vi "Load New Launcher.vi"(7 "Plugin Loader Path Override":path, 8 "error in (no error)":errorcluster, 9 "Loader Name Override":string, 10 "Loader Load Info":T1, 11 "CIFPluginManager in":refnum<class "CIFPluginManager.lvclass">) -> (0 "error out":errorcluster)   [LabVIEW 2021, in "CIFPluginManager.lvclass"]
uses:
  CIFPluginManager.lvclass
  typedef/Loader Load Command.ctl
  typedef/Loader Type.ctl
  CIFPluginManager.lvclass/CIFPluginManager.ctl
  <vilib>/CIF Foundation/CIF Core/CIFUtilities/CIFConfigurationFile/typedef/Location Type.ctl
  <vilib>/CIF Foundation/CIF Core/CIFCore/Common/Typedef/Errors.ctl
  <vilib>/CIF Foundation/CIF Core/CIFUtilities/CIFConfigurationFile/CIF Configuration File Location.vi
  <vilib>/CIF Foundation/CIF Utilities/Errors/Append Error Location.vi
  <vilib>/CIF Foundation/CIF Utilities/Time/System Time/LabVIEW Time to TAI Time.vi
  Engine Launch/CIF Engine Launch.lvlib
  <vilib>/CIF Foundation/CIF Utilities/Time/Time_CIF_U.lvlib
  <vilib>/CIF Foundation/CIF Core/CIFUtilities/CIFConfigurationFile/CIF Configuration File.lvlib
  <vilib>/CIF Foundation/CIF Core/CIFCore/Common/CIFCoreCommon.lvlib
  <vilib>/CIF Foundation/CIF Core/CIFUtilities/CIFLogs/CIFLogs.lvlib
  <vilib>/CIF Foundation/CIF Core/CIFUtilities/CIFLogs/Typedef/Message Type.ctl
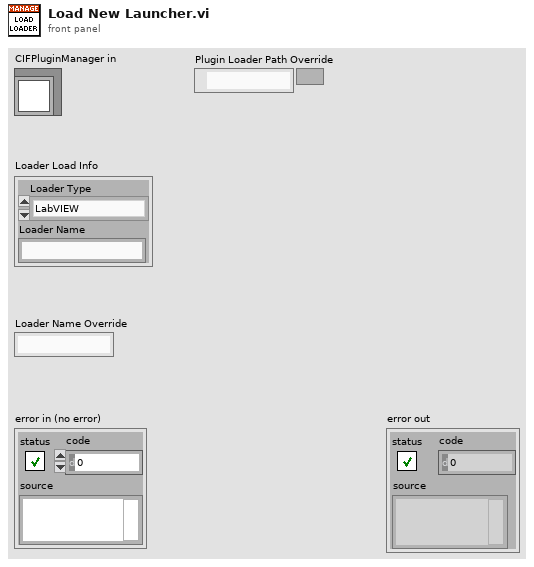
[diagram p1: front panel]
types:
  T1 = typedef "CIFPluginManager.lvclass/Loader Load Command.ctl" = cluster{"Loader Type":T2, "Loader Name":string}
  T2 = typedef "CIFPluginManager.lvclass/Loader Type.ctl" = enum16{"LabVIEW"}
  T3 = typedef "CIFPluginManager.lvclass/Loader Map.ctl" = map{string, T4}
  T4 = typedef "CIFPluginManager.lvclass/Loaders.ctl" = cluster{"Loader Type":T2, "grpc_port":i32, "pid":u32, "gRPC ID":T5, "Load Timestamp":i64, "Unloading":bool, "Ready for removal":bool, "Unload Timestamp":i64}
  T5 = typedef "grpc-lvsupport-release.lvlib/grpcId.ctl" = u64
  T6 = typedef "CIFCoreCommon.lvlib/Errors.ctl" = enum16{"Invalid Clock ID", "Long Sleep", "gRPC Server Not Found", "Config Parse", "Timestamp Wrap", "Delayed Execution", "Duplicate Channel", "Missing Channel", "Incorrect Type", "Flatten Error", "Unflatten Data", "Unique Name", "Plugin Not Found", "Plugin Type Not Found", "Plugin Version Not Found", "Manager Not Found", "Numerical Issue", "Time Jump", "Clock ID Match", "Channel Length", "Plugin Connection", "gRPC Server Connection", "PPL Name Match", "Build", "Config Log Parse", "Plugin Load", "UI Subpanel Load", "Python Name", "Invalid Name", "Unable to Change Ch Buffer", "Failed Kill", "Failed SysExec", "Function Not Implemented", "Load Timeout", "Invalid FTE", "Manager Crash"}
  T7 = typedef "CIF Configuration File.lvlib/Location Type.ctl" = enum16{"Config File", "Manager", "Protos", "Plugins", "UI Plugins", "Logs", "Orchestrations", "Loaders"}
  T8 = typedef "CIFLogs.lvlib/Message Type.ctl" = enum16{"Error", "Information", "Print Terminal", "Configuration"}
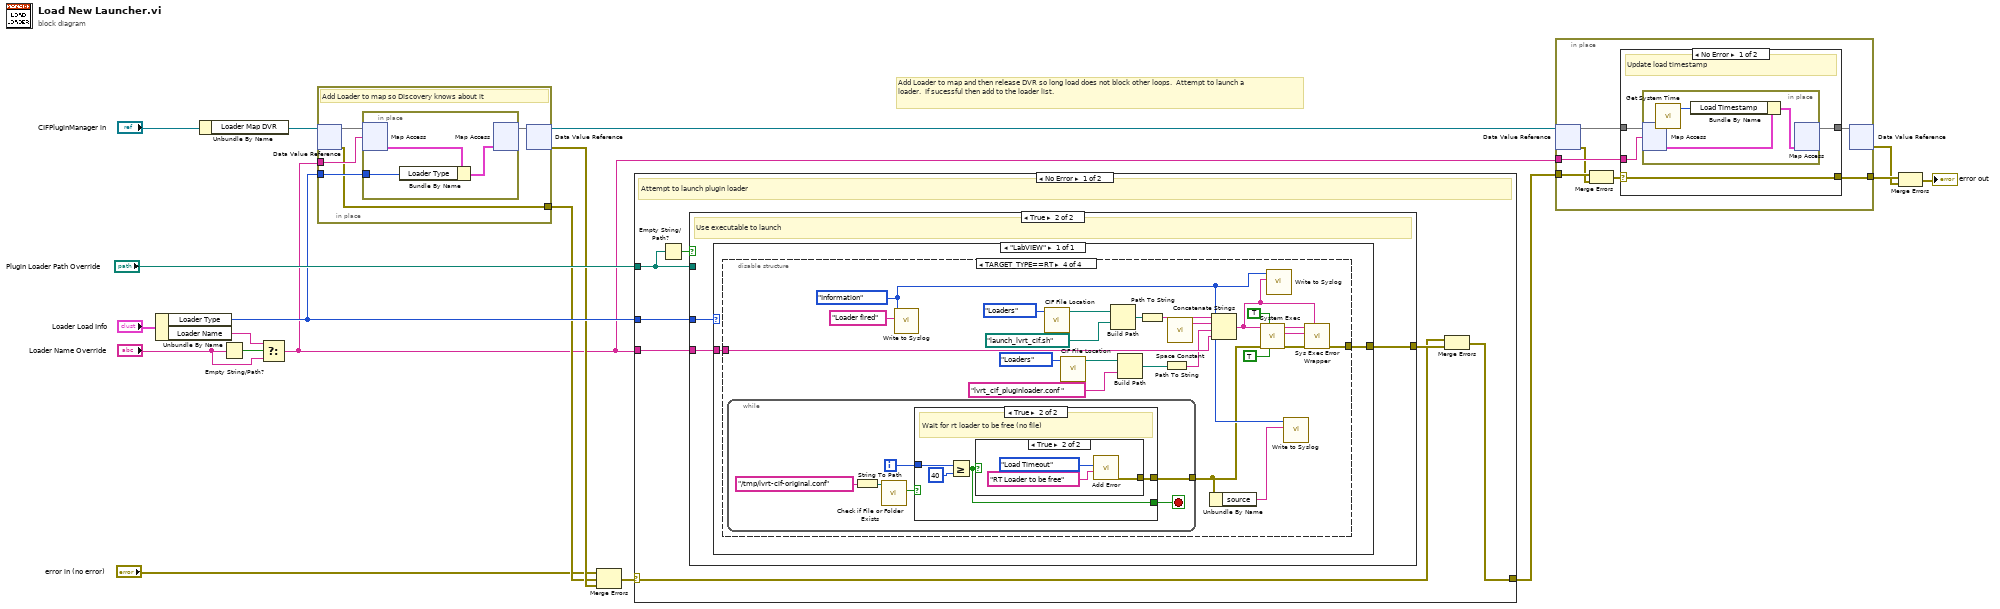
[diagram p0: block diagram]
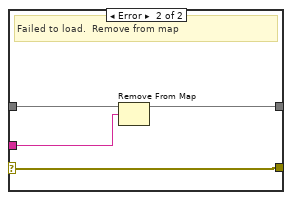
[diagram p2: hidden frame]
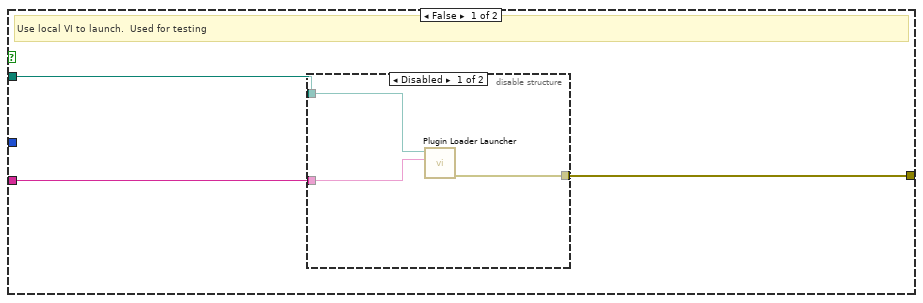
[diagram p3: hidden frame]
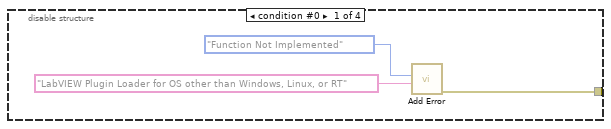
[diagram p5: hidden frame]
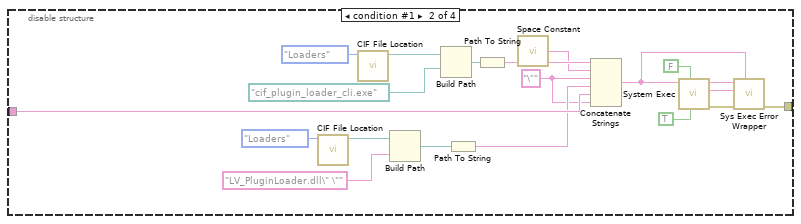
[diagram p6: hidden frame]
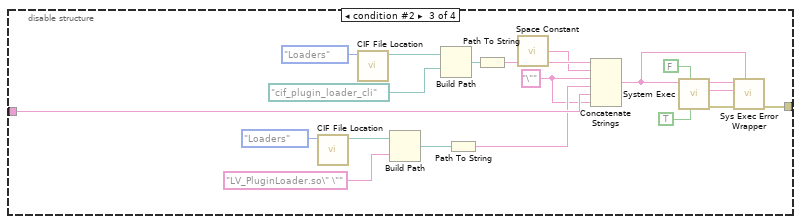
[diagram p7: hidden frame]
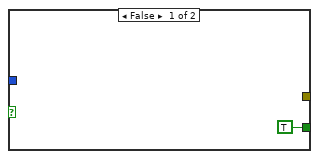
[diagram p8: hidden frame]
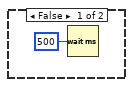
[diagram p9: hidden frame]
diagram:
  # "Add Loader to map and then release DVR so long load does not block other loops.  Attempt to launch a loader.  If sucessful then add to the loader list."
  n1 = Unbundle By Name("Loader Load Info") -> ("Loader Type"=w11:T2, "Loader Name"=w14:string)
  n2 = Unbundle By Name("CIFPluginManager in") -> ("Loader Map DVR"=w12:refnum<data-value>)
  n3 = Empty String/Path?(string/path="Loader Name Override") -> (empty?=w16:bool)
  n4 = Select(t=w14, s=w16, f="Loader Name Override") -> (s? t:f=w3:string)
  n5 = in-place {
    in-place-border: w3 -> [w22]
    in-place-border: w11 -> [w21]
    in-place-border: [w19] -> w9
    # "Add Loader to map so Discovery knows about it"
    n6 = in-place-dvr #1(w12) -> (w23:T3, w19:errorcluster)
    n7 = in-place {
      in-place-border: w21 -> [w25]
      n8 = in-place-map #2(w23, w22) -> (w26:T4)  [unwired: 1 in, 1 out]
      n9 = Bundle By Name(cluster=w26, "Loader Type"=w25) -> (w24:T4)
      n10 = in-place-map #2(w24) -> (w20:T3)  [unwired: 1 in, 2 out]
    }
    n11 = in-place-dvr #1(w20) -> (w8:refnum<data-value>, w10:errorcluster)
  }
  n12 = Merge Errors("error in (no error)", w9, w10) -> (w1:errorcluster)
  n13 = case shown="No Error" w1 {
    selector: w1 -> [w31 w126]
    tunnel: [w27 w126] -> w7
    tunnel: "Plugin Loader Path Override" -> [w30 _]
    tunnel: w3 -> [w28 _]
    tunnel: w11 -> [w33 _]
    frame No Error {
      # "Attempt to launch plugin loader"
      n14 = Empty String/Path?(string/path=w30) -> (empty?=w29:bool)
      n15 = case shown="True" w29 {
        tunnel: w30 -> [w36 _]
        tunnel: [w35 w41] -> w32
        tunnel: w28 -> [w34 w42]
        tunnel: w33 -> [_ w40]
        frame False {
          # "Use local VI to launch.  Used for testing"
          n16 = disable-structure shown="Disabled" {
            disable-tunnel: w36 -> [w39 _]
            disable-tunnel: [w38 _] -> w35
            disable-tunnel: w34 -> [w37 _]
            frame Disabled {
              n17 = call "Plugin Loader Launcher.vi"("Loader Name Override"=w37, "Plugin Loader Path Override"=w39) -> ("error out"=w38:errorcluster)  [unwired: 9 in]
            }
            frame Enabled {
            }
          }
        }
        frame True {
          # "Use executable to launch"
          n18 = case shown="\"LabVIEW\"" w40 {
            tunnel: w42 -> [w44]
            tunnel: [w43] -> w41
            frame "LabVIEW" {
              n19 = disable-structure shown="TARGET_TYPE==RT" {
                disable-tunnel: w44 -> [_ w57 w77 w100]
                disable-tunnel: [w47 w51 w71 w95] -> w43
                frame condition #0 {
                  n20 = call <vilib>:"Add Error.vi"("String to Append"="LabVIEW Plugin Loader for OS other than Windows, Linux, or RT", "Error"=Errors."Function Not Implemented") -> ("error out"=w47:errorcluster)  [unwired: 9 in]
                }
                frame condition #1 {
                  w53 = "\"" ("Loader Name Override")
                  n21 = call <vilib>:"CIF File Location.vi"("LocationType"=Location_Type."Loaders") -> ("Location"=w59:path)  [unwired: 10 in]
                  n22 = call <vilib>:"CIF File Location.vi"("LocationType"=Location_Type."Loaders") -> ("Location"=w63:path)  [unwired: 10 in]
                  n23 = Build Path(base path=w59, name or relative path="LV_PluginLoader.dll\" \"" ("Loader Name Override")) -> (appended path=w56:path)
                  n24 = Build Path(base path=w63, name or relative path=path "cif_plugin_loader_cli.exe") -> (appended path=w67:path)
                  n25 = Path To String(path=w56) -> (string=w55:string)
                  n26 = Path To String(path=w67) -> (string=w66:string)
                  n27 = call <vilib>:"Space Constant.vi"() -> ("String"=w54:string)
                  n28 = Concatenate Strings(w66, w54, w53, w55, w57, w53) -> (w48:string)
                  n29 = call <vilib>:"System Exec.vi"("run minimized? (F)"=TRUE, "wait until completion? (T)"=FALSE, "command line"=w48) -> ("error out"=w52:errorcluster, "standard error"=w50:string, "standard output"=w49:string)  [unwired: 5 in, 1 out]
                  n30 = call <vilib>:"Sys Exec Error Wrapper.vi"("command line"=w48, "error in (no error)"=w52, "standard error"=w50, "standard output"=w49) -> ("error out"=w51:errorcluster)  [unwired: 7 in]
                }
                frame condition #2 {
                  w73 = "\"" ("Loader Name Override")
                  n31 = call <vilib>:"CIF File Location.vi"("LocationType"=Location_Type."Loaders") -> ("Location"=w79:path)  [unwired: 10 in]
                  n32 = call <vilib>:"CIF File Location.vi"("LocationType"=Location_Type."Loaders") -> ("Location"=w83:path)  [unwired: 10 in]
                  n33 = Build Path(base path=w79, name or relative path="LV_PluginLoader.so\" \"" ("Loader Name Override")) -> (appended path=w76:path)
                  n34 = Build Path(base path=w83, name or relative path=path "cif_plugin_loader_cli") -> (appended path=w87:path)
                  n35 = Path To String(path=w76) -> (string=w75:string)
                  n36 = Path To String(path=w87) -> (string=w86:string)
                  n37 = call <vilib>:"Space Constant.vi"() -> ("String"=w74:string)
                  n38 = Concatenate Strings(w86, w74, w73, w75, w77, w73) -> (w68:string)
                  n39 = call <vilib>:"System Exec.vi"("run minimized? (F)"=TRUE, "wait until completion? (T)"=FALSE, "command line"=w68) -> ("error out"=w72:errorcluster, "standard error"=w70:string, "standard output"=w69:string)  [unwired: 5 in, 1 out]
                  n40 = call <vilib>:"Sys Exec Error Wrapper.vi"("command line"=w68, "error in (no error)"=w72, "standard error"=w70, "standard output"=w69) -> ("error out"=w71:errorcluster)  [unwired: 7 in]
                }
                frame condition #3 (active) {
                  w90 = Message_Type."Information" ("CIF Message Type")
                  n41 = while {
                    tunnel: [w112] -> w89
                    i -> [w111]
                    stop <- w113 stop-if-true
                    n42 = String To Path(string="/tmp/lvrt-cif-original.conf" ("Loader Name Override")) -> (path=w116:path)
                    n43 = call <vilib>:"Check if File or Folder Exists.vi"("path"=w116) -> ("file or folder exists?"=w114:bool)  [unwired: 8 in, 2 out]
                    n44 = case shown="True" w114 {
                      tunnel: [_ w121] -> w112
                      tunnel: w111 -> [_ w118]
                      tunnel: [TRUE w119] -> w113
                      frame False {
                      }
                      frame True {
                        # "Wait for rt loader to be free (no file)"
                        n45 = Greater Or Equal?(x=w118, y=40) -> (x >= y?=w119:bool)
                        n46 = case shown="True" w119 {
                          tunnel: [_ w123] -> w121
                          frame False {
                            n47 = Wait (ms)(milliseconds to wait=u32 500) -> ()  [unwired: 1 out]
                          }
                          frame True {
                            n48 = call <vilib>:"Add Error.vi"("String to Append"="RT Loader to be free", "Error"=Errors."Load Timeout") -> ("error out"=w123:errorcluster)  [unwired: 9 in]
                          }
                        }
                      }
                    }
                  }
                  n49 = call <vilib>:"Write to Syslog.vi"("message"="Loader fired", "CIF Message Type"=w90) -> ()  [unwired: 9 in, 1 out]
                  n50 = call <vilib>:"CIF File Location.vi"("LocationType"=Location_Type."Loaders") -> ("Location"=w106:path)  [unwired: 10 in]
                  n51 = call <vilib>:"CIF File Location.vi"("LocationType"=Location_Type."Loaders") -> ("Location"=w102:path)  [unwired: 10 in]
                  n52 = Build Path(base path=w106, name or relative path=path "launch_lvrt_cif.sh") -> (appended path=w110:path)
                  n53 = Build Path(base path=w102, name or relative path="lvrt_cif_pluginloader.conf " ("Loader Name Override")) -> (appended path=w99:path)
                  n54 = Path To String(path=w110) -> (string=w109:string)
                  n55 = Path To String(path=w99) -> (string=w98:string)
                  n56 = call <vilib>:"Space Constant.vi"() -> ("String"=w97:string)
                  n57 = Unbundle By Name(w89) -> ("source"=w88:string)
                  n58 = Concatenate Strings(w109, w97, w98, w100) -> (w91:string)
                  n59 = call <vilib>:"System Exec.vi"("run minimized? (F)"=TRUE, "wait until completion? (T)"=TRUE, "error in (no error)"=w89, "command line"=w91) -> ("error out"=w96:errorcluster, "standard error"=w94:string, "standard output"=w93:string)  [unwired: 4 in, 1 out]
                  n60 = call <vilib>:"Write to Syslog.vi"("message"=w91, "CIF Message Type"=w90) -> ()  [unwired: 9 in, 1 out]
                  n61 = call <vilib>:"Write to Syslog.vi"("message"=w88, "CIF Message Type"=w90) -> ()  [unwired: 9 in, 1 out]
                  n62 = call <vilib>:"Sys Exec Error Wrapper.vi"("command line"=w91, "error in (no error)"=w96, "standard error"=w94, "standard output"=w93) -> ("error out"=w95:errorcluster)  [unwired: 7 in]
                }
              }
            }
          }
        }
      }
      n63 = Merge Errors(w31, w32) -> (w27:errorcluster)
    }
    frame Error {
      # "Error adding to map"
    }
  }
  n64 = in-place {
    in-place-border: w3 -> [w133]
    in-place-border: w7 -> [w130]
    in-place-border: [w127] -> w6
    n65 = in-place-dvr #3(w8) -> (w132:T3, w128:errorcluster)
    n66 = Merge Errors(w130, w128) -> (w129:errorcluster)
    n67 = case shown="No Error" w129 {
      selector: w129 -> [w134 w141]
      tunnel: w133 -> [w137 w143]
      tunnel: w132 -> [w136 w144]
      tunnel: [w135 w142] -> w131
      tunnel: [w134 w141] -> w127
      frame No Error {
        # "Update load timestamp"
        n68 = in-place {
          # "Update load timestamp"
          n69 = in-place-map #4(w136, w137) -> (w140:T4)  [unwired: 1 in, 1 out]
          n70 = call <vilib>:"Get System Time.vi"() -> ("Time (ns)"=w139:i64)  [unwired: 5 in]
          n71 = Bundle By Name(cluster=w140, "Load Timestamp"=w139) -> (w138:T4)
          n72 = in-place-map #4(w138) -> (w135:T3)  [unwired: 1 in, 2 out]
        }
      }
      frame Error {
        # "Failed to load.  Remove from map"
        n73 = Remove From Map(10:w143, 11:w144) -> (3:w142:T3)  [unwired: 2 out]
      }
    }
    n74 = in-place-dvr #3(w131) -> (w5:errorcluster)  [unwired: 1 out]
  }
  n75 = Merge Errors(w6, w5) -> (→"error out":errorcluster)
